vi "GetNamedSemaphorePrefix.vi"() -> (2 "Named Semaphore Prefix":string)   [LabVIEW 2020]
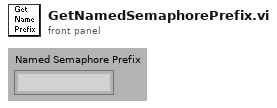
[diagram p1: front panel]
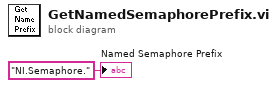
[diagram p0: block diagram]
diagram:
  "Named Semaphore Prefix" <- "NI.Semaphore." ("Named Semaphore Prefix")
